vi "File.Rotate.Perform Rotation.vi"(8 "error in (no error)":errorcluster, 11 "File.Rotate in":refnum<class "File.Rotate.lvclass">) -> (0 "error out":errorcluster, 1 "Next Check(s)":dbl, 2 "Task Status":T1(array[cluster]), 3 "File.Rotate out":refnum<class "File.Rotate.lvclass">)   [LabVIEW 2024, in "EQMF.lvlib" / "File Utils.lvlib" / "File.Rotate.lvclass"]
uses:
  File.Rotate.lvclass
  File.Rotate.lvclass/File.Rotate.ctl
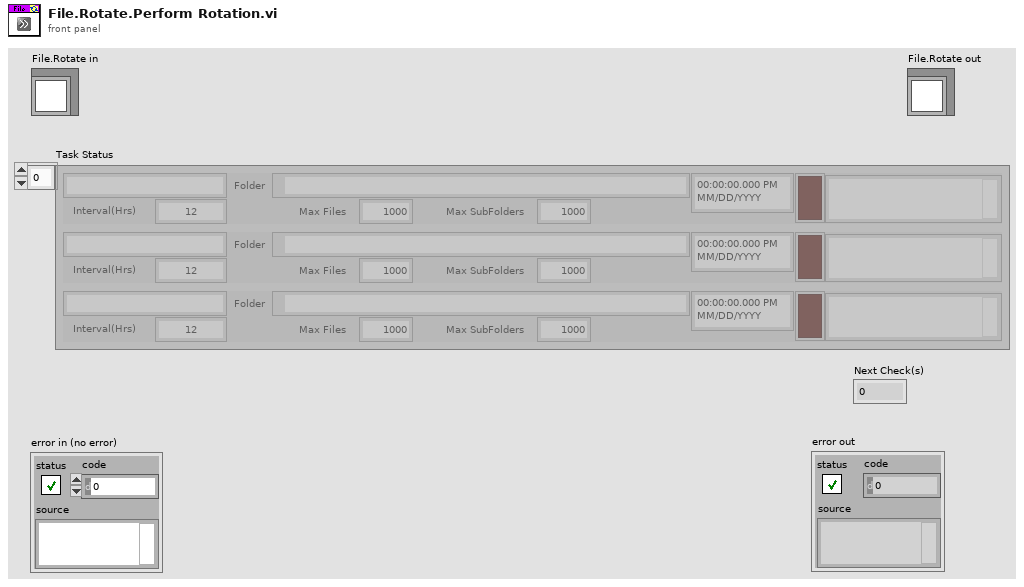
[diagram p1: front panel]
types:
  T1 = cluster{"Name":string, "Interval":dbl, "Folder":path, "Max Files":i32, "Max SubFolders":i32, "LastRotate":timestamp, "Error":bool, "Status":string}[]
  T2 = typedef "EQMF.lvlib/File Utils.lvlib/File.Rotate.lvclass/File.Rotate.Rotation Task Item.ctl" = cluster{"Name":string, "Interval":dbl, "Folder":path, "Max Files":i32, "Max SubFolders":i32, "LastRotate":timestamp, "Error":bool, "Status":string}
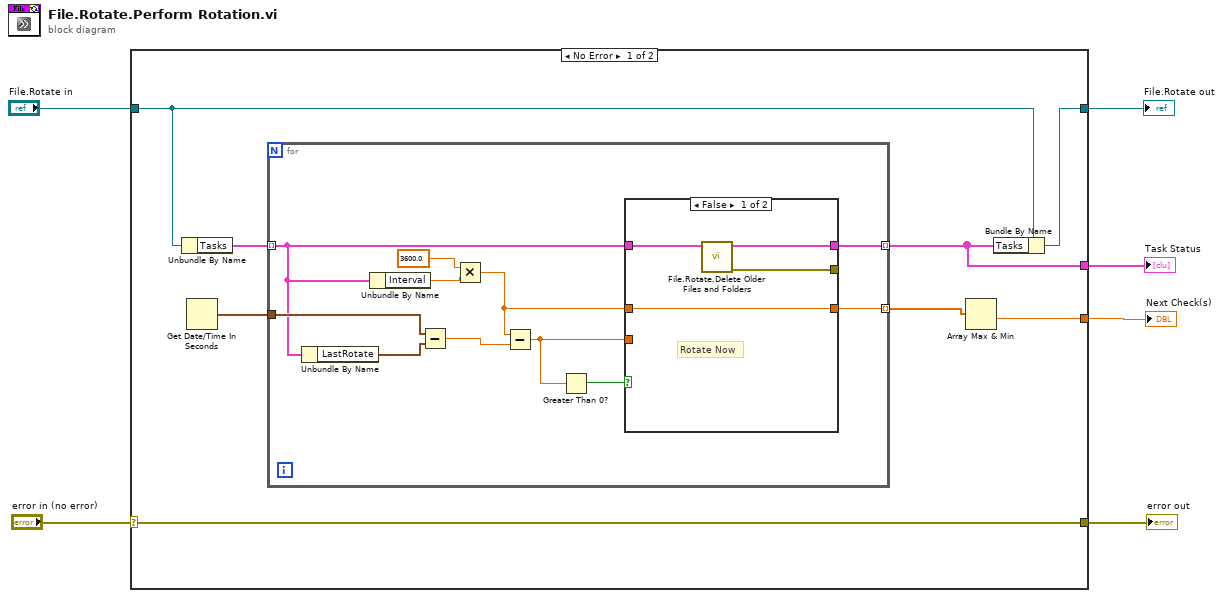
[diagram p0: block diagram]
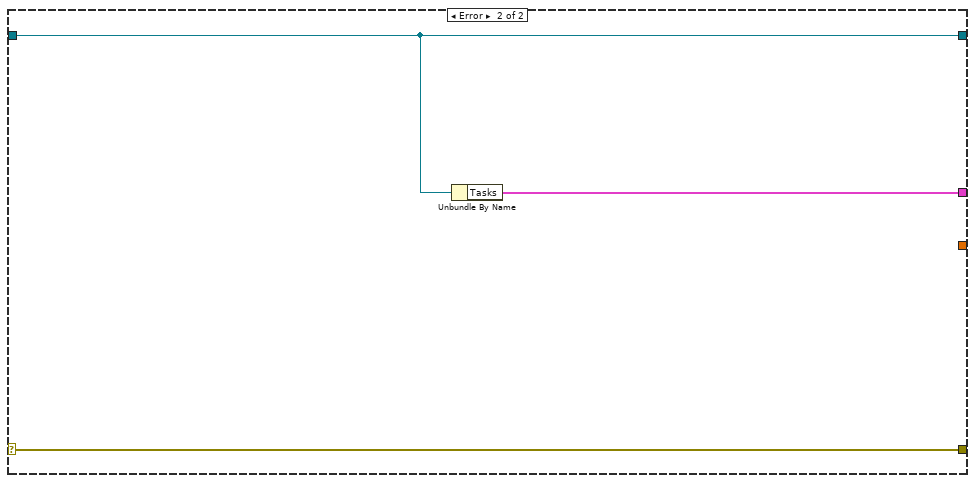
[diagram p3: hidden frame]
diagram:
  n1 = case shown="No Error" "error in (no error)" {
    selector: "error in (no error)" -> [w14 w34]
    tunnel: [w14 w34] -> w5
    tunnel: [w11 w33] -> w3
    tunnel: "File.Rotate in" -> [w10 w33]
    tunnel: [w9 w32] -> w2
    tunnel: [w7 _] -> w1
    frame No Error {
      n2 = Unbundle By Name(w10) -> ("Tasks"=w13:T2[])
      n3 = Get Date/Time In Seconds() -> (seconds since 1Jan1904=w12:timestamp)
      n4 = for {
        tunnel: w13 -> [w21] mode=indexing
        tunnel: w12 -> [w24]
        tunnel: [w20] -> w9 mode=indexing
        tunnel: [w19] -> w8 mode=indexing
        n5 = Unbundle By Name(w21) -> ("LastRotate"=w25:timestamp)
        n6 = Unbundle By Name(w21) -> ("Interval"=w17:dbl)
        n7 = Subtract(x=w24, y=w25) -> (x-y=w15:dbl)
        n8 = Multiply(x=3600.0 ("y"), y=w17) -> (x*y=w16:dbl)
        n9 = Subtract(x=w16, y=w15) -> (x-y=w22:dbl)
        n10 = Greater Than 0?(x=w22) -> (x > 0?=w23:bool)
        n11 = case shown="False" w23 {
          tunnel: w22 -> [_ w31]
          tunnel: w16 -> [w26 _]
          tunnel: w21 -> [w29 w30]
          tunnel: [w28 w30] -> w20
          tunnel: [w27 _] -> _
          tunnel: [w26 w31] -> w19
          frame False {
            # "Rotate Now"
            n12 = call "File.Rotate.Delete Older Files and Folders.vi"("Task"=w29) -> ("error out"=w27:errorcluster, "Task Out"=w28:T2)  [unwired: 9 in]
          }
          frame True {
            # "Sched Rotation"
          }
        }
      }
      n13 = Array Max & Min(array=w8) -> (min value=w7:dbl)  [unwired: 3 out]
      n14 = Bundle By Name(cluster=w10, "Tasks"=w9) -> (w11:refnum<class "File.Rotate.lvclass">)
    }
    frame Error {
      n15 = Unbundle By Name(w33) -> ("Tasks"=w32:T2[])
    }
  }
  "error out" <- w5
  "File.Rotate out" <- w3
  "Task Status" <- w2
  "Next Check(s)" <- w1
